vi "test1-ResponseWithError.vi"(8 "error in (no error)":errorcluster, 11 "TestCase in":refnum<class "testcase-CSMResponse.lvclass">) -> (0 "error out":errorcluster, 3 "TestCase out":refnum<class "testcase-CSMResponse.lvclass">)   [LabVIEW 2017, in "testcase-CSMResponse.lvclass"]
uses:
  testcase-CSMResponse.lvclass
  68a58439-6a05-4de0-8ad5-cfc0558cbd3a.vi
  src/user.lib/_NEVSTOP/Communicable State Machine(CSM)/AdvanceAPI/CSM - Make String Arguments Safe.vi
  src/user.lib/_NEVSTOP/Communicable State Machine(CSM)/AdvanceAPI/CSM - Keywords.vi
  <vilib>/addons/_JKI Toolkits/VI Tester/TestCase.llb/TestCase.lvclass
  src/user.lib/_NEVSTOP/Communicable State Machine(CSM)/Communicable State Machine.lvlib
  C:/Program Files (x86)/National Instruments/LabVIEW 2017/vi.lib/addons/_JKI Toolkits/VI Tester/TestCase.llb/TestCase.lvclass
panel:
  out "concatenated string":string
  out "Loopcount":i32
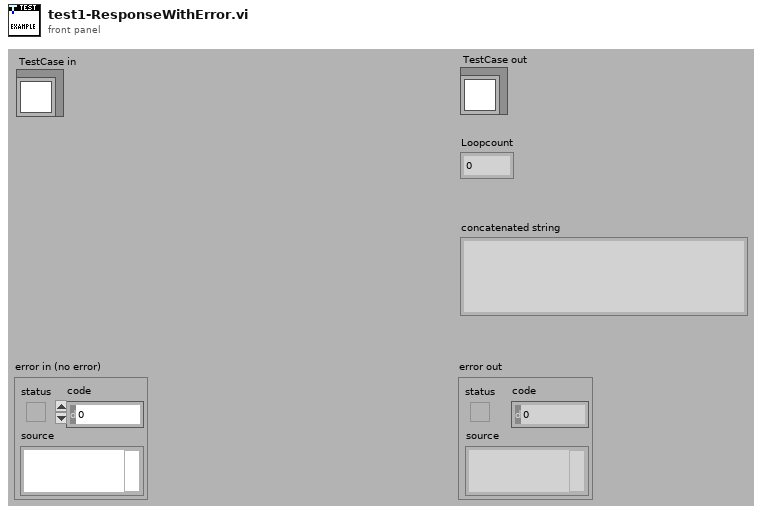
[diagram p1: front panel]
types:
  T1 = cluster{"Arguments":string, "Response":string, "error":errorcluster}
  T2 = cluster{"status":bool, "code":bool, "source":bool}
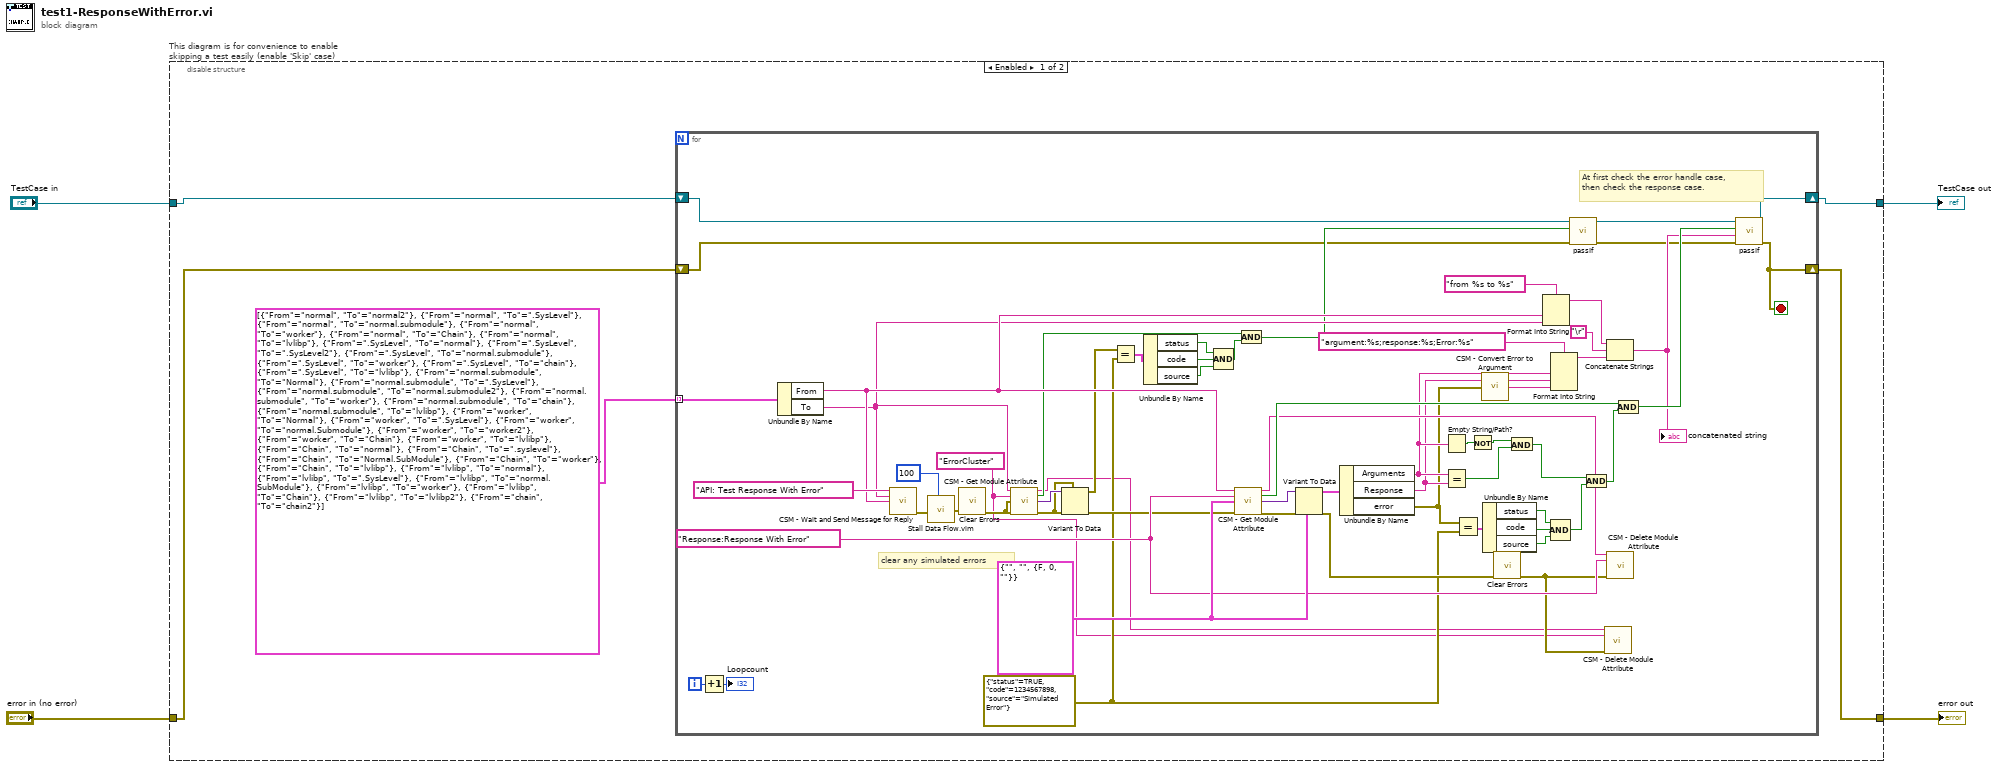
[diagram p0: block diagram]
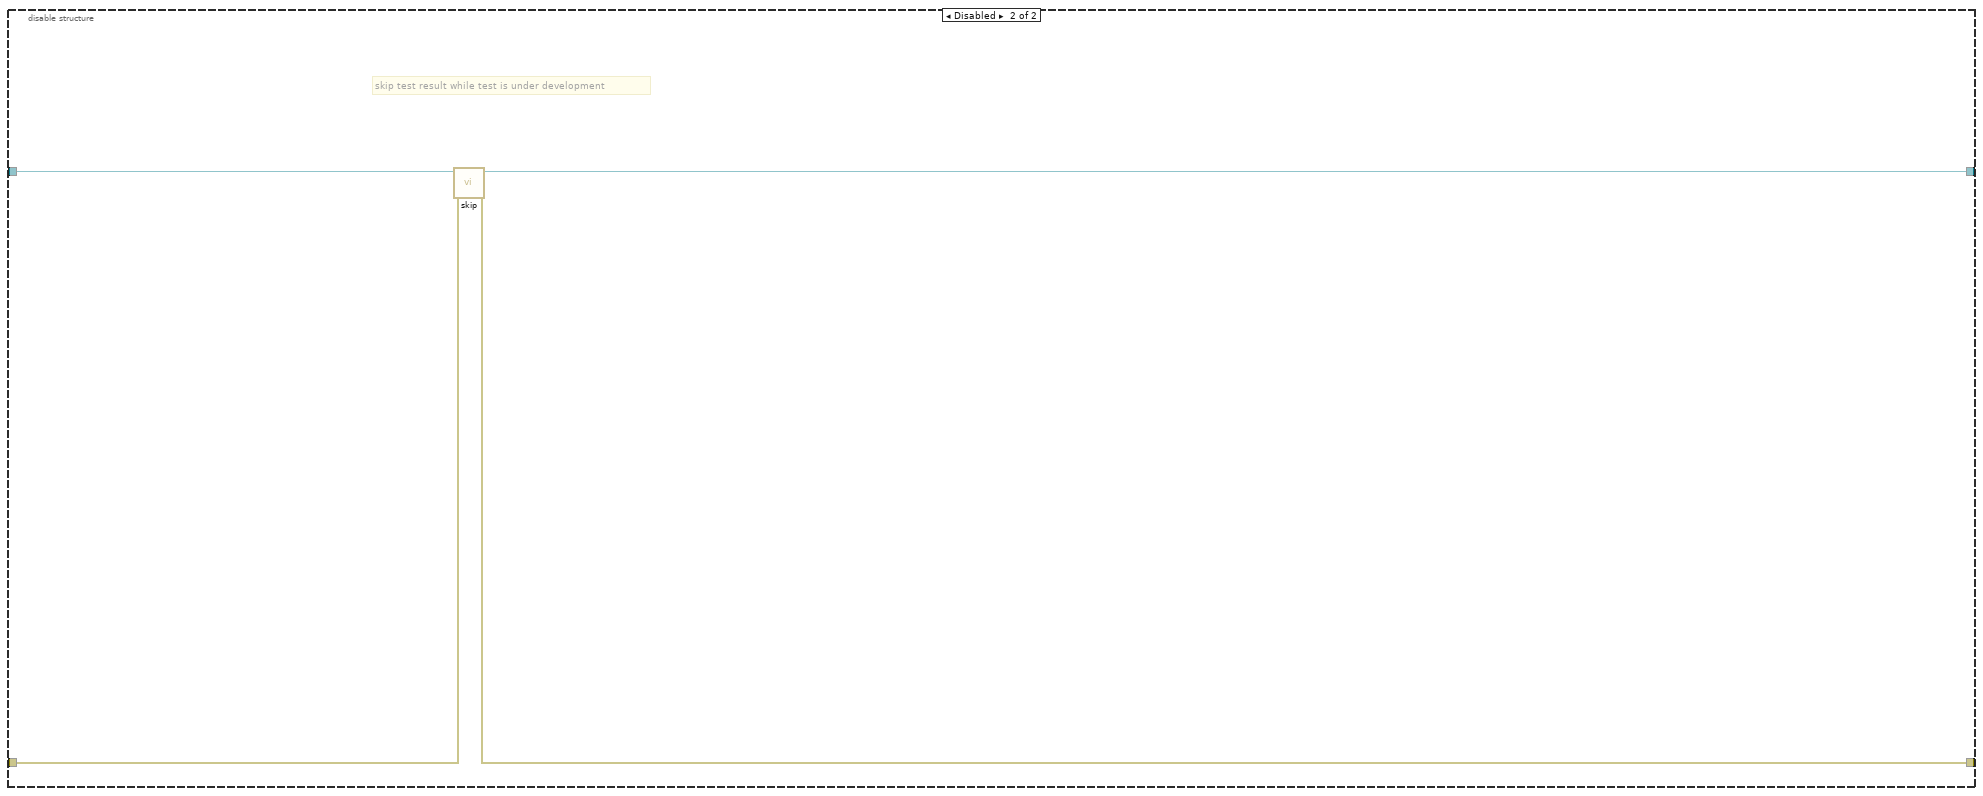
[diagram p2: hidden frame]
diagram:
  n1 = disable-structure "This diagram is for convenience to enable skipping a test easily (enable 'Skip' case)" shown="Enabled" {
    disable-tunnel: "TestCase in" -> [w9 w73]
    disable-tunnel: [w8 w71] -> w1
    disable-tunnel: [w7 w72] -> w3
    disable-tunnel: "error in (no error)" -> [w6 w70]
    frame Enabled {
      n2 = for {
        tunnel: cluster{"From":string, "To":string}[] [{"From"="normal", "To"="normal2"}, {"From"="normal", "To"=".SysLevel"}, {"From"="normal", "To"="normal.submodule"}, {"From"="normal", "To"="worker"}, {"From"="normal", "To"="Chain"}, {"From"="normal", "To"="lvlibp"}, {"From"=".SysLevel", "To"="normal"}, {"From"=".SysLevel", "To"=".SysLevel2"}, {"From"=".SysLevel", "To"="normal.submodule"}, {"From"=".SysLevel", "To"="worker"}, {"From"=".SysLevel", "To"="chain"}, {"From"=".SysLevel", "To"="lvlibp"}, {"From"="normal.submodule", "To"="Normal"}, {"From"="normal.submodule", "To"=".SysLevel"}, {"From"="normal.submodule", "To"="normal.submodule2"}, {"From"="normal.submodule", "To"="worker"}, {"From"="normal.submodule", "To"="chain"}, {"From"="normal.submodule", "To"="lvlibp"}, {"From"="worker", "To"="Normal"}, {"From"="worker", "To"=".SysLevel"}, {"From"="worker", "To"="normal.Submodule"}, {"From"="worker", "To"="worker2"}, {"From"="worker", "To"="Chain"}, {"From"="worker", "To"="lvlibp"}, {"From"="Chain", "To"="normal"}, {"From"="Chain", "To"=".syslevel"}, {"From"="Chain", "To"="Normal.SubModule"}, {"From"="Chain", "To"="worker"}, {"From"="Chain", "To"="lvlibp"}, {"From"="lvlibp", "To"="normal"}, {"From"="lvlibp", "To"=".SysLevel"}, {"From"="lvlibp", "To"="normal.SubModule"}, {"From"="lvlibp", "To"="worker"}, {"From"="lvlibp", "To"="Chain"}, {"From"="lvlibp", "To"="lvlibp2"}, {"From"="chain", "To"="chain2"}] -> [w60] mode=indexing
        shift-right: [w69] -> w8
        shift-left: w9 -> [w14]
        shift-right: [w43] -> w7
        shift-left: w6 -> [w16]
        i -> [w35]
        stop <- w43 stop-if-true
        w10 = "ErrorCluster" ("Attribute")
        w23 = errorcluster {"status"=TRUE, "code"=1234567898, "source"="Simulated Error"} ("error out")
        w66 = T1 {"Arguments"="", "Response"="", "error"={"status"=FALSE, "code"=0, "source"=""}}
        w57 = "Response:Response With Error" ("State")
        # "At first check the error handle case,\nthen check the response case."
        # "clear any simulated errors"
        n3 = Increment(x=w35) -> (x+1=→"Loopcount":i32)
        n4 = Unbundle By Name(w60) -> ("From"=w36:string, "To"=w30:string)
        n5 = call "CSM - Wait and Send Message for Reply.vi"("State"="API: Test Response With Error", "Arguments (\"\")"=w30, "Target Module"=w36) -> ("error out"=w33:errorcluster)  [unwired: 10 in, 2 out]
        n6 = call "Stall Data Flow.vim"("value in"=w33, "milliseconds to wait"=u32 100) -> ("value out"=w32:errorcluster)  [unwired: 1 out]
        n7 = call <vilib>:"Clear Errors.vi"("error in (no error)"=w32) -> ("error out"=w29:errorcluster)  [unwired: 5 in, 1 out]
        n8 = call "CSM - Get Module Attribute.vi"("CSM Name"=w30, "Attribute"=w10, "Default Value (Empty Variant)"=w29, "Error In"=w29) -> ("CSM Name (Dup)"=w11:string, "Found"=w28:bool, "Value"=w26:variant, "error out"=w25:errorcluster)  [unwired: 7 in, 1 out]
        n9 = Variant To Data(error in=w25, type=w25, Variant=w26) -> (data=w24:errorcluster, error out=w27:errorcluster)
        n10 = Equal?(x=w24, y=w23) -> (x = y?=w19:T2)
        n11 = Unbundle By Name(w19) -> ("status"=w20:bool, "code"=w21:bool, "source"=w22:bool)
        n12 = Compound Arithmetic op=AND(w20, w21, w22) -> (w18:bool)
        n13 = call "CSM - Get Module Attribute.vi"("CSM Name"=w36, "Attribute"=w57, "Default Value (Empty Variant)"=w66, "Error In"=w27) -> ("CSM Name (Dup)"=w58:string, "Found"=w63:bool, "Value"=w65:variant, "error out"=w67:errorcluster)  [unwired: 7 in, 1 out]
        n14 = And(x=w28, y=w18) -> (x .and. y?=w17:bool)
        n15 = Variant To Data(error in=w67, type=w66, Variant=w65) -> (data=w64:T1, error out=w44:errorcluster)
        n16 = Unbundle By Name(w64) -> ("Arguments"=w52:string, "Response"=w51:string, "error"=w42:errorcluster)
        n17 = Empty String/Path?(string/path=w52) -> (empty?=w56:bool)
        n18 = Equal?(x=w52, y=w51) -> (x = y?=w54:bool)
        n19 = Equal?(x=w42, y=w23) -> (x = y?=w41:T2)
        n20 = Not(x=w56) -> (.not. x?=w55:bool)
        n21 = call "CSM - Convert Error to Argument.vi"("Error"=w42) -> ("Argument"=w50:string)  [unwired: 4 in]
        n22 = Unbundle By Name(w41) -> ("status"=w40:bool, "code"=w39:bool, "source"=w38:bool)
        n23 = call <vilib>:"Clear Errors.vi"("error in (no error)"=w44) -> ("error out"=w12:errorcluster)  [unwired: 5 in, 1 out]
        n24 = And(x=w55, y=w54) -> (x .and. y?=w53:bool)
        n25 = Format Into String(format string="from %s to %s", w36, w30) -> (resulting string=w46:string)  [unwired: 2 in, 1 out]
        n26 = Format Into String(format string="argument:%s;response:%s;Error:%s", w52, w51, w50) -> (resulting string=w49:string)  [unwired: 2 in, 1 out]
        n27 = Compound Arithmetic op=AND(w40, w39, w38) -> (w37:bool)
        n28 = call-dynamic "passIf.vi"("error in (no error)"=w16, "pass"=w17, "TestCase in"=w14) -> ("error out"=w15:errorcluster, "TestCase out"=w13:refnum<class "testcase-CSMResponse.lvclass">)  [unwired: 7 in]
        n29 = And(x=w53, y=w37) -> (x .and. y?=w62:bool)
        n30 = call "CSM - Delete Module Attribute.vi"("CSM Name"=w11, "Attribute"=w10, "Error In"=w12) -> ()  [unwired: 9 in, 4 out]
        n31 = Concatenate Strings(w46, "\r", w49) -> (w47:string)
        "concatenated string" <- w47
        n32 = call "CSM - Delete Module Attribute.vi"("CSM Name"=w58, "Attribute"=w57, "Error In"=w12) -> ()  [unwired: 9 in, 4 out]
        n33 = And(x=w63, y=w62) -> (x .and. y?=w61:bool)
        n34 = call-dynamic "passIf.vi"("error in (no error)"=w15, "message (\"\")"=w47, "pass"=w61, "TestCase in"=w13) -> ("error out"=w43:errorcluster, "TestCase out"=w69:refnum<class "testcase-CSMResponse.lvclass">)  [unwired: 6 in]
      }
    }
    frame Disabled {
      # "skip test result while test is under development"
      n35 = call <vilib>:"skip.vi"("error in (no error)"=w70, "TestCase in"=w73) -> ("error out"=w72:errorcluster, "TestCase out"=w71:refnum<class "testcase-CSMResponse.lvclass">)  [unwired: 8 in]
    }
  }
  "error out" <- w3
  "TestCase out" <- w1
